vi "create.Time.vi"(8 "error in":errorcluster, 10 "Time.Parameters":T1, 11 "Time in":refnum<class "Time.lvclass">) -> (0 "error out":errorcluster, 3 "Time out":refnum<class "Time.lvclass">)   [LabVIEW 2020, in "Time.lvclass"]
uses:
  Time.lvclass
  Time.Parameters.ctl
  FieldSpec.ctl
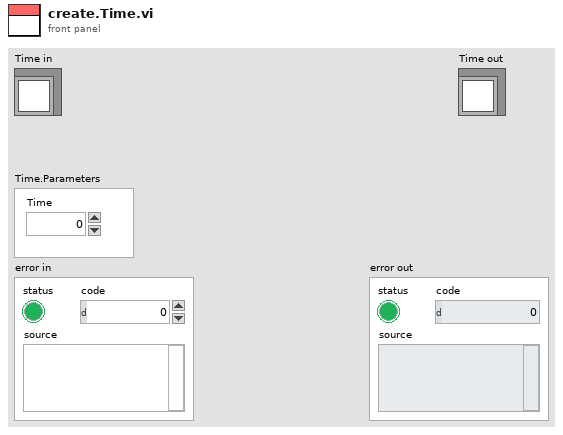
[diagram p1: front panel]
types:
  T1 = typedef "Time.lvclass/Time.Parameters.ctl" = cluster{"Time":u32}
  T2 = typedef "FieldSpec.ctl" = cluster{"Name":string, "Offset":i32, "Length":i32, "FieldType":enum16{"Alphanumeric", "Binary", "BinaryLongPrice", "BinaryShortPrice", "BitField", "PrintableAscii", "Value"}, "FieldValue":variant}
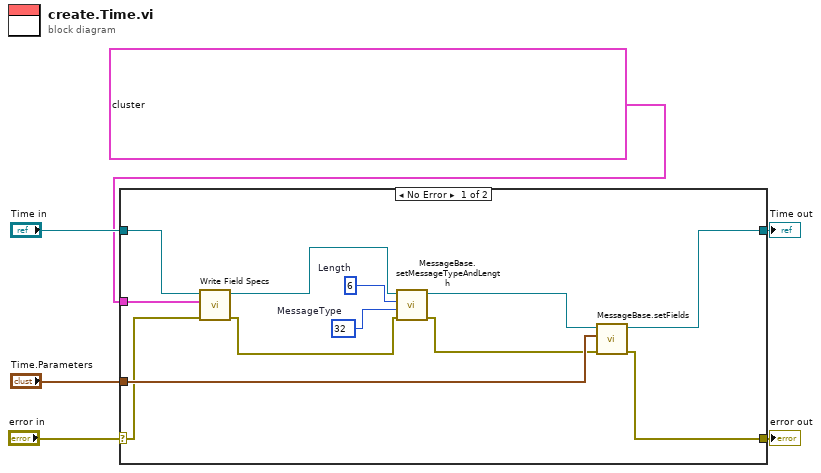
[diagram p0: block diagram]
diagram:
  n1 = case shown="No Error" "error in" {
    selector: "error in" -> [w8 w20]
    tunnel: [w10 w20] -> w1
    tunnel: [w11 w19] -> w5
    tunnel: "Time in" -> [w13 w19]
    tunnel: T2[] [{"Name"="Length", "Offset"=0, "Length"=1, "FieldType"=enum."Binary", "FieldValue"=variant}, {"Name"="MessageType", "Offset"=1, "Length"=1, "FieldType"=enum."Value", "FieldValue"=variant}, {"Name"="Time", "Offset"=2, "Length"=4, "FieldType"=enum."Binary", "FieldValue"=variant}] ("appended array") -> [w14 _]
    tunnel: "Time.Parameters" -> [w9 _]
    frame No Error {
      w18 = u8 32  # MessageType
      w17 = u8 6  # Length
      n2 = call-dynamic "Write Field Specs.vi"("error in (no error)"=w8, "Field Specs"=w14, "MessageBase in"=w13) -> ("error out"=w16:errorcluster, "MessageBase out"=w15:refnum<class "Time.lvclass">)  [unwired: 7 in]
      n3 = call-dynamic "MessageBase.setMessageTypeAndLength.vi"("error in (no error)"=w16, "MessageType"=w18, "Length"=w17, "MessageBase in"=w15) -> ("error out"=w7:errorcluster, "MessageBase out"=w12:refnum<class "Time.lvclass">)  [unwired: 6 in]
      n4 = call-dynamic "MessageBase.setFields.vi"("error in (no error)"=w7, "Cluster (dup)"=w9, "MessageBase in"=w12) -> ("error out"=w10:errorcluster, "MessageBase out"=w11:refnum<class "Time.lvclass">)  [unwired: 7 in]
    }
    frame Error {
    }
  }
  "Time out" <- w5
  "error out" <- w1
